vi "Init Data.vi"(8 "error in (no error)":errorcluster, 11 "Rigol DG822 Square in":refnum<class "Rigol DG822 Square.lvclass">) -> (0 "error out":errorcluster, 3 "Rigol DG822 Square out":refnum<class "Rigol DG822 Square.lvclass">)   [LabVIEW 2021, in "Rigol DG822 UI.lvlib" / "Rigol DG822 Square.lvlib" / "Rigol DG822 Square.lvclass"]
uses:
  Rigol DG822 Square.lvclass
  Rigol DG822 Square.lvclass/Rigol DG822 Square.ctl
  General/Files/lvlibp/Actors.lvlibp/Actors/Actors/Actors.lvclass
  D:/LabVIEW/General/Files/lvlibp/Actors.lvlibp/Actors/Actors/Actors.lvclass
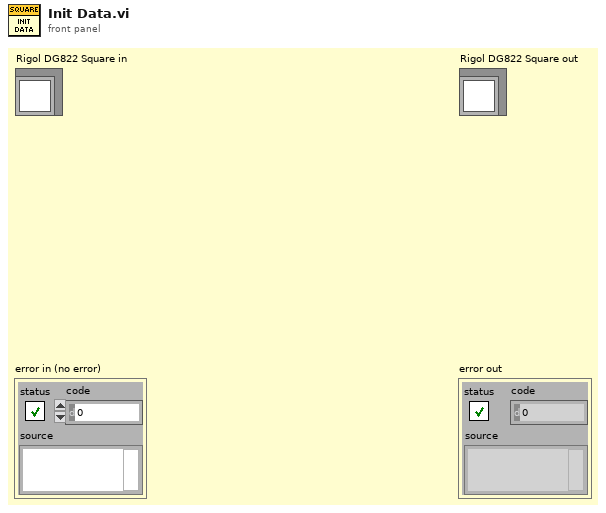
[diagram p1: front panel]
types:
  T1 = cluster{"Freq-Period":string, "Freq-Period 2":string, "Freq-Period 3":string, "Freq-Period 4":string, "Freq-Period 5":string}
  T2 = cluster{"Control Label 5":string, "Control Label 6":string, "Control Label":string, "Control Label 2":string, "Control Label 3":string, "Control Label 4":string}
  T3 = cluster{"Control Label":string, "Control Label 2":string, "Control Label 3":string}
  T4 = typedef "FT Controls Cluster.ctl" = cluster{"Freq/Period":bool, "Ampl/HighL":bool, "Offset/LowL":bool, "Duty/Width":bool}
  T5 = typedef "String Indicators Cluster.ctl" = cluster{"Freq-Period":string, "Ampl-HighL":string, "Offset-LowL":string, "Phase":string, "Duty-Width":string, "RisEdge":string, "FallEdge":string}
  T6 = enum32{"No Selection", "MHz", "kHz", "Hz", "mHz", "uHz"}
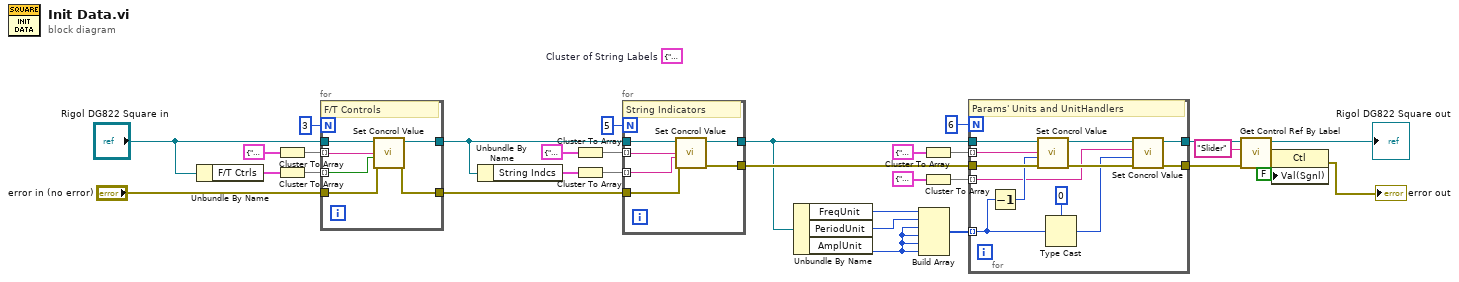
[diagram p0: block diagram]
diagram:
  (unwired) T1 {"Freq-Period"="String Indcs.Freq-Period", "Freq-Period 2"="String Indcs.Ampl-HighL", "Freq-Period 3"="String Indcs.Offset-LowL", "Freq-Period 4"="String Indcs.Phase", "Freq-Period 5"="String Indcs 2.Duty"}  # Cluster of String Labels
  n1 = Unbundle By Name("Rigol DG822 Square in") -> ("F/T Ctrls"=w28:T4)
  n2 = Cluster To Array(cluster=T3 {"Control Label"="F/T Ctrls.Freq/Period", "Control Label 2"="F/T Ctrls.Ampl/HighL", "Control Label 3"="F/T Ctrls.Offset/LowL"}) -> (array=w26:string[])
  n3 = Cluster To Array(cluster=w28) -> (array=w25:bool[])
  n4 = for {
    N: 3 -> [_]
    tunnel: w26 -> [w39] mode=indexing
    tunnel: "Rigol DG822 Square in" -> [w38]
    tunnel: w25 -> [w37] mode=indexing
    tunnel: "error in (no error)" -> [w36]
    tunnel: [w35] -> w22
    tunnel: [w34] -> w18
    # "F/T Controls"
    n5 = call "Set Concrol Value.vi"("error in (no error)"=w36, "Value"=w37, "Control Label"=w39, "Actors in"=w38) -> ("error out"=w35:errorcluster, "Actors out"=w34:refnum<class "Rigol DG822 Square.lvclass">)  [unwired: 6 in]
  }
  n6 = Unbundle By Name(w18) -> ("String Indcs"=w21:T5)
  n7 = Cluster To Array(cluster=T1 {"Freq-Period"="String Indcs.Freq-Period", "Freq-Period 2"="String Indcs.Ampl-HighL", "Freq-Period 3"="String Indcs.Offset-LowL", "Freq-Period 4"="String Indcs.Phase", "Freq-Period 5"="String Indcs 2.Duty"} ("Cluster of String Labels")) -> (array=w19:string[])
  n8 = Cluster To Array(cluster=w21) -> (array=w20:string[])
  n9 = for {
    N: 5 -> [_]
    tunnel: w19 -> [w45] mode=indexing
    tunnel: w18 -> [w44]
    tunnel: w20 -> [w43] mode=indexing
    tunnel: w22 -> [w42]
    tunnel: [w41] -> w16
    tunnel: [w40] -> w14
    # "String Indicators"
    n10 = call "Set Concrol Value.vi"("error in (no error)"=w42, "Value"=w43, "Control Label"=w45, "Actors in"=w44) -> ("error out"=w41:errorcluster, "Actors out"=w40:refnum<class "Rigol DG822 Square.lvclass">)  [unwired: 6 in]
  }
  n11 = Unbundle By Name(w14) -> ("FreqUnit"=w13:T6, "PeriodUnit"=w11:enum32{"No Selection", "s", "ms", "us", "ns"}, "AmplUnit"=w12:enum32{"No Selection", "Vpp", "mVpp"})
  n12 = Build Array(w13, w11, w12, w12, w12, w12) -> (w15:u32[])
  n13 = Cluster To Array(cluster=T2 {"Control Label 5"="FreqUnitHandler", "Control Label 6"="PeriodUnitHandler", "Control Label"="AmplUnitHandler", "Control Label 2"="HighLUnitHandler", "Control Label 3"="OffsetUnitHandler", "Control Label 4"="LowLUnitHandler"}) -> (array=w31:string[])
  n14 = Cluster To Array(cluster=T2 {"Control Label 5"="FreqUnit", "Control Label 6"="PeriodUnit", "Control Label"="AmplUnit", "Control Label 2"="HighLUnit", "Control Label 3"="OffsetUnit", "Control Label 4"="LowLUnit"}) -> (array=w29:string[])
  n15 = for {
    N: 6 -> [_]
    tunnel: w14 -> [w56]
    tunnel: [w54] -> w3
    tunnel: [w53] -> w1
    tunnel: w16 -> [w52]
    tunnel: w31 -> [w51] mode=indexing
    tunnel: w29 -> [w49] mode=indexing
    tunnel: w15 -> [w46] mode=indexing
    # "Params' Units and UnitHandlers"
    n16 = Decrement(x=w46) -> (x-1=w50:u32)
    n17 = call "Set Concrol Value.vi"("error in (no error)"=w52, "Value"=w50, "Control Label"=w51, "Actors in"=w56) -> ("error out"=w57:errorcluster, "Actors out"=w55:refnum<class "Rigol DG822 Square.lvclass">)  [unwired: 6 in]
    n18 = Type Cast(type=0, x=w46) -> (*(type *) &x=w48:i32)
    n19 = call "Set Concrol Value.vi"("error in (no error)"=w57, "Value"=w48, "Control Label"=w49, "Actors in"=w55) -> ("error out"=w53:errorcluster, "Actors out"=w54:refnum<class "Rigol DG822 Square.lvclass">)  [unwired: 6 in]
  }
  n20 = call "Get Control Ref By Label.vi"("error in (no error)"=w1, "Control Label"="Slider", "Actors in"=w3) -> ("error out"=w7:errorcluster, "Control Ref"=w6:refnum<vi>, "Actors out"=→"Rigol DG822 Square out":refnum<class "Rigol DG822 Square.lvclass">)  [unwired: 6 in]
  n21 = property class="Ctl"(reference=w6, error in=w7, "Val(Sgnl)"=FALSE) -> (error out=→"error out":errorcluster)  [unwired: 1 out]
